vi "Divide.vi"(1 "x":sgl, 2 "y":sgl, 4 "Divider3":refnum<class "Divider3.lvclass">) -> (6 "x/y":sgl)   [LabVIEW 2017, in "Divider3.lvclass"]
uses:
  Divider3.lvclass
  Divider.lvclass
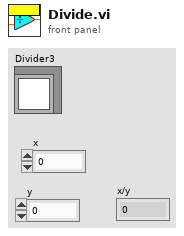
[diagram p1: front panel]
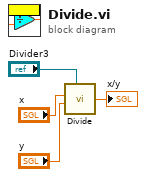
[diagram p0: block diagram]
diagram:
  n1 = call-parent "Divide.vi"("x"="x", "y"="y", "Divider"="Divider3") -> ("x/y"=→"x/y":sgl)  [unwired: 4 in]
